vi "niSwitch DMM-array.vi"() -> ()   [LabVIEW 2011]
doc: "I. Description:\n\nThis example demonstrates how to scan a series of channels on a switch module and take measurements with an NI digital multimeter using handshaking. \n\nHANDSHAKING:\nFirst, the DMM is initiated and waits for a digital pulse from the switch before taking any measurements. When the switch scanning task is started, it connects the first channel in its scan list, waits for the channel to settle and generates a digital pulse-Scan Advanced. When the DMM receives this digital pulse, it takes the first measurement and generates a digital pulse-Measurement Complete (MC). When the switch receives this digital pulse, it advances to the next entry in its scan list and this continues.\n\nII. Instructions for Running:\n\nTo make this example work with your switch, complete the following:\nSWITCH SETUP: (refer to the NI Switches Help) \nEnter the DAQmx/traditional DAQ switch resource name.\nSelect the correct topology for your switch module.\nEnter a valid scan list.\nSelect valid values for Trigger Input and Scan Advanced Output. \n\nDMM SETUP: (refer to your NI DMM documentation)\nEnter the DAQmx/traditional DAQ DMM resource name.\nSelect measurement type, range and resolution.\nEnter number of samples.\nSelect a valid Measurement Complete Destination and Trigger Source.\n\nRefer to the NI Switches Help to determine if your switch supports scanning, the scan list syntax, and the valid channel names and valid resource names for your switch module.\n\nIII. Block Diagram Steps:\n\nA) The switch is configured first. Triggers and scan list are set. The scanning configuration is downloaded to the hardware with niSwitch Commit.vi.\nB) The DMM is configured. Functions, range, resolution, triggers and number of points to take are set. When the DMM initiates, it configures its hardware according to the settings and waits for a trigger. \nC) When the switch initiates it connects the first channels in its scan list, waits for the relays to settle and send its Scan Advanced signal to trigger the DMM for its first measurement. Once the DMM has taken a measurement, the DMM sends its MC signal to the switch to advance to the next entry in the scan list. \nD) The DMM returns to the user the number of measurements specified in \"Samples to Fetch at a Time\". When the stop button is pushed the acquisition stops.\nE) Terminates the scanning operation, closes the session to the switch, and displays errors if any.\n\nIV. I/O Connections Overview:\n\nRefer to the NI Switches Getting Started Guide and NI Switches Help for information about connecting signals to your switch module."
uses:
  <instrlib>/niDMM/nidmm.llb/niDMM Function.ctl
  <instrlib>/niSwitch/niSwitch.LLB/niSwitch Topologies.ctl
  <instrlib>/niDMM/nidmm.llb/niDMM Trigger.ctl
  <instrlib>/niDMM/nidmm.llb/niDMM Sample Trigger.ctl
  <vilib>/Utility/NIReport.llb/NI_report.lvclass
  <instrlib>/niDMM/nidmm.llb/niDMM Configure Measurement Absolute.vi
  <vilib>/addons/_office/excel.llb/Excel Easy Table (str).vi
  <vilib>/addons/_office/NI_ReportGenerationToolkit.lvlib
  <vilib>/Utility/NIReport.llb/Excel/NI_Excel.lvclass
panel:
  in  "自低向高色码表":u32[](array[colorbox])=[16860, 5898160, 6745856, 16765184, 16711680]
  out "转置的数组":dbl[][](array[numeric])=[[0.49997470177871867, 0.4999905131670195, 0.4999715395010585, 0.5000284604989416, 0.49999367544467965, 0.5000158113883009, 0.4999873508893593, 0.5, 0.5, 0.499981026334039], [0.5000031622776602, 0.5000126491106407, 0.49997470177871867, 0.4999715395010585, 0.5, 0.5000252982212814, 0.5000031622776602, 0.4999905131670195, 0.49997786405637884, 0.5], [0.5, 0.499981026334039, 0.4999905131670195, 0.5000221359436212, 0.49997470177871867, 0.5000126491106407, 0.49999367544467965, 0.5000221359436212, 0.5000221359436212, 0.499981026334039], [0.5000158113883009, 0.5000252982212814, 0.5000284604989416, 0.4999905131670195, 0.5000284604989416, 0.5000284604989416, 0.5000063245553203, 0.49998418861169913, 0.49998418861169913, 0.5000252982212814], [0.5000221359436212, 0.49997470177871867, 0.49997470177871867, 0.5, 0.5, 0.49997786405637884, 0.5000031622776602, 0.5000063245553203, 0.5000158113883009, 0.500018973665961], [0.4999873508893593, 0.5000063245553203, 0.5000284604989416, 0.49997786405637884, 0.4999715395010585, 0.499981026334039, 0.5000126491106407, 0.49999367544467965, 0.499981026334039, 0.4999968377223398], [0.5000252982212814, 0.5000158113883009, 0.5000158113883009, 0.5000094868329805, 0.4999968377223398, 0.5000221359436212, 0.5000126491106407, 0.5000221359436212, 0.5, 0.4999873508893593], [0.5, 0.500018973665961, 0.49997470177871867, 0.5000094868329805, 0.499981026334039, 0.49998418861169913, 0.49997470177871867, 0.49997470177871867, 0.5000094868329805, 0.5000126491106407], [0.4999873508893593, 0.49998418861169913, 0.5000284604989416, 0.5000126491106407, 0.5000094868329805, 0.5000284604989416, 0.49999367544467965, 0.5, 0.5000221359436212, 0.49999367544467965], [0.500018973665961, 0.4999968377223398, 0.5000221359436212, 0.5000094868329805, 0.5000094868329805, 0.5000031622776602, 0.5000126491106407, 0.49997470177871867, 0.5000158113883009, 0.5000063245553203]]
  in  "选项卡控件":enum32{"强度图", "数据"}(tab)
  in  "Enum":enum16{"最大值", "最小值"}(ring)
  out "强度极限图":dbl[][](graph)=[[0.49997470177871867, 0.4999905131670195, 0.4999715395010585, 0.5000284604989416, 0.49999367544467965, 0.5000158113883009, 0.4999873508893593, 0.5, 0.5, 0.499981026334039], [0.5000031622776602, 0.5000126491106407, 0.49997470177871867, 0.4999715395010585, 0.5, 0.5000252982212814, 0.5000031622776602, 0.4999905131670195, 0.49997786405637884, 0.5], [0.5, 0.499981026334039, 0.4999905131670195, 0.5000221359436212, 0.49997470177871867, 0.5000126491106407, 0.49999367544467965, 0.5000221359436212, 0.5000221359436212, 0.499981026334039], [0.5000158113883009, 0.5000252982212814, 0.5000284604989416, 0.4999905131670195, 0.5000284604989416, 0.5000284604989416, 0.5000063245553203, 0.49998418861169913, 0.49998418861169913, 0.5000252982212814], [0.5000221359436212, 0.49997470177871867, 0.49997470177871867, 0.5, 0.5, 0.49997786405637884, 0.5000031622776602, 0.5000063245553203, 0.5000158113883009, 0.500018973665961], [0.4999873508893593, 0.5000063245553203, 0.5000284604989416, 0.49997786405637884, 0.4999715395010585, 0.499981026334039, 0.5000126491106407, 0.49999367544467965, 0.499981026334039, 0.4999968377223398], [0.5000252982212814, 0.5000158113883009, 0.5000158113883009, 0.5000094868329805, 0.4999968377223398, 0.5000221359436212, 0.5000126491106407, 0.5000221359436212, 0.5, 0.4999873508893593], [0.5, 0.500018973665961, 0.49997470177871867, 0.5000094868329805, 0.499981026334039, 0.49998418861169913, 0.49997470177871867, 0.49997470177871867, 0.5000094868329805, 0.5000126491106407], [0.4999873508893593, 0.49998418861169913, 0.5000284604989416, 0.5000126491106407, 0.5000094868329805, 0.5000284604989416, 0.49999367544467965, 0.5, 0.5000221359436212, 0.49999367544467965], [0.500018973665961, 0.4999968377223398, 0.5000221359436212, 0.5000094868329805, 0.5000094868329805, 0.5000031622776602, 0.5000126491106407, 0.49997470177871867, 0.5000158113883009, 0.5000063245553203]]
  out "强度图":dbl[][](graph)=[[0.49997470177871867, 0.4999905131670195, 0.4999715395010585, 0.5000284604989416, 0.49999367544467965, 0.5000158113883009, 0.4999873508893593, 0.5, 0.5, 0.499981026334039], [0.5000031622776602, 0.5000126491106407, 0.49997470177871867, 0.4999715395010585, 0.5, 0.5000252982212814, 0.5000031622776602, 0.4999905131670195, 0.49997786405637884, 0.5], [0.5, 0.499981026334039, 0.4999905131670195, 0.5000221359436212, 0.49997470177871867, 0.5000126491106407, 0.49999367544467965, 0.5000221359436212, 0.5000221359436212, 0.499981026334039], [0.5000158113883009, 0.5000252982212814, 0.5000284604989416, 0.4999905131670195, 0.5000284604989416, 0.5000284604989416, 0.5000063245553203, 0.49998418861169913, 0.49998418861169913, 0.5000252982212814], [0.5000221359436212, 0.49997470177871867, 0.49997470177871867, 0.5, 0.5, 0.49997786405637884, 0.5000031622776602, 0.5000063245553203, 0.5000158113883009, 0.500018973665961], [0.4999873508893593, 0.5000063245553203, 0.5000284604989416, 0.49997786405637884, 0.4999715395010585, 0.499981026334039, 0.5000126491106407, 0.49999367544467965, 0.499981026334039, 0.4999968377223398], [0.5000252982212814, 0.5000158113883009, 0.5000158113883009, 0.5000094868329805, 0.4999968377223398, 0.5000221359436212, 0.5000126491106407, 0.5000221359436212, 0.5, 0.4999873508893593], [0.5, 0.500018973665961, 0.49997470177871867, 0.5000094868329805, 0.499981026334039, 0.49998418861169913, 0.49997470177871867, 0.49997470177871867, 0.5000094868329805, 0.5000126491106407], [0.4999873508893593, 0.49998418861169913, 0.5000284604989416, 0.5000126491106407, 0.5000094868329805, 0.5000284604989416, 0.49999367544467965, 0.5, 0.5000221359436212, 0.49999367544467965], [0.500018973665961, 0.4999968377223398, 0.5000221359436212, 0.5000094868329805, 0.5000094868329805, 0.5000031622776602, 0.5000126491106407, 0.49997470177871867, 0.5000158113883009, 0.5000063245553203]]
  out "Measurements":dbl[](array[numeric])=[0.499981026334039, 0.5, 0.499981026334039, 0.5000252982212814, 0.500018973665961, 0.4999968377223398, 0.4999873508893593, 0.5000126491106407, 0.49999367544467965, 0.5000063245553203, 0.5, 0.49997786405637884, 0.5000221359436212, 0.49998418861169913, 0.5000158113883009, 0.499981026334039, 0.5, 0.5000094868329805, 0.5000221359436212, 0.5000158113883009, 0.5, 0.4999905131670195, 0.5000221359436212, 0.49998418861169913, 0.5000063245553203, 0.49999367544467965, 0.5000221359436212, 0.49997470177871867, 0.5, 0.49997470177871867, 0.4999873508893593, 0.5000031622776602, 0.49999367544467965, 0.5000063245553203, 0.5000031622776602, 0.5000126491106407, 0.5000126491106407, 0.49997470177871867, 0.49999367544467965, 0.5000126491106407, 0.5000158113883009, 0.5000252982212814, 0.5000126491106407, 0.5000284604989416, 0.49997786405637884, 0.499981026334039, 0.5000221359436212, 0.49998418861169913, 0.5000284604989416, 0.5000031622776602, 0.49999367544467965, 0.5, 0.49997470177871867, 0.5000284604989416, 0.5, 0.4999715395010585, 0.4999968377223398, 0.499981026334039, 0.5000094868329805, 0.5000094868329805, 0.5000284604989416, 0.4999715395010585, 0.5000221359436212, 0.4999905131670195, 0.5, 0.49997786405637884, 0.5000094868329805, 0.5000094868329805, 0.5000126491106407, 0.5000094868329805, 0.4999715395010585, 0.49997470177871867, 0.4999905131670195, 0.5000284604989416, 0.49997470177871867, 0.5000284604989416, 0.5000158113883009, 0.49997470177871867, 0.5000284604989416, 0.5000221359436212, 0.4999905131670195, 0.5000126491106407, 0.499981026334039, 0.5000252982212814, 0.49997470177871867, 0.5000063245553203, 0.5000158113883009, 0.500018973665961, 0.49998418861169913, 0.4999968377223398, 0.49997470177871867, 0.5000031622776602, 0.5, 0.5000158113883009, 0.5000221359436212, 0.4999873508893593, 0.5000252982212814, 0.5, 0.4999873508893593, 0.500018973665961] caption="原始数据" format="%.7f"
  out "输出数组":dbl[][](array[numeric])=[[0.499981026334039, 0.5, 0.499981026334039, 0.5000252982212814, 0.500018973665961, 0.4999968377223398, 0.4999873508893593, 0.5000126491106407, 0.49999367544467965, 0.5000063245553203], [0.5, 0.49997786405637884, 0.5000221359436212, 0.49998418861169913, 0.5000158113883009, 0.499981026334039, 0.5, 0.5000094868329805, 0.5000221359436212, 0.5000158113883009], [0.5, 0.4999905131670195, 0.5000221359436212, 0.49998418861169913, 0.5000063245553203, 0.49999367544467965, 0.5000221359436212, 0.49997470177871867, 0.5, 0.49997470177871867], [0.4999873508893593, 0.5000031622776602, 0.49999367544467965, 0.5000063245553203, 0.5000031622776602, 0.5000126491106407, 0.5000126491106407, 0.49997470177871867, 0.49999367544467965, 0.5000126491106407], [0.5000158113883009, 0.5000252982212814, 0.5000126491106407, 0.5000284604989416, 0.49997786405637884, 0.499981026334039, 0.5000221359436212, 0.49998418861169913, 0.5000284604989416, 0.5000031622776602], [0.49999367544467965, 0.5, 0.49997470177871867, 0.5000284604989416, 0.5, 0.4999715395010585, 0.4999968377223398, 0.499981026334039, 0.5000094868329805, 0.5000094868329805], [0.5000284604989416, 0.4999715395010585, 0.5000221359436212, 0.4999905131670195, 0.5, 0.49997786405637884, 0.5000094868329805, 0.5000094868329805, 0.5000126491106407, 0.5000094868329805], [0.4999715395010585, 0.49997470177871867, 0.4999905131670195, 0.5000284604989416, 0.49997470177871867, 0.5000284604989416, 0.5000158113883009, 0.49997470177871867, 0.5000284604989416, 0.5000221359436212], [0.4999905131670195, 0.5000126491106407, 0.499981026334039, 0.5000252982212814, 0.49997470177871867, 0.5000063245553203, 0.5000158113883009, 0.500018973665961, 0.49998418861169913, 0.4999968377223398], [0.49997470177871867, 0.5000031622776602, 0.5, 0.5000158113883009, 0.5000221359436212, 0.4999873508893593, 0.5000252982212814, 0.5, 0.4999873508893593, 0.500018973665961]]
  in  "error in (no error)":errorcluster caption="错误输入（无错误）"
  in  "Save":bool caption="Stop"
  out "大小":i32=100
  in  "通道个数":i32=100 min=9 max=100
  in  "最大采集时间 (毫秒)":i32=5000
  in  "topology name":T1="2530/1-Wire Dual 64x1 Mux" caption="拓扑名称"
  in  "measurement type":T2=enum."DC Current" caption="测量类型"
  in  "range":dbl=0.5 caption="范围" format="%.2f"
  in  "resolution":dbl=1e-05 caption="分辨率" format="%.0p"
  in  "resource name":refnum<k15>="4071" caption="万用表名称"
  in  "scan list":string="ch0->com0&ch64->com4;ch1->com0&ch64->com4;ch2->com0&ch64->com4;ch3->com0&ch64->com4;ch4->com0&ch64->com4;ch5->com0&ch64->com4;ch6->com0&ch64->com4;ch7->com0&ch64->com4;ch8->com0&ch64->com4;ch9->com0&ch64->com4;ch0->com0&ch65->com4;ch1->com0&ch65->com4;ch2->com0&ch65->com4;ch3->com0&ch65->com4;ch4->com0&ch65->com4;ch5->com0&ch65->com4;ch6->com0&ch65->com4;ch7->com0&ch65->com4;ch8->com0&ch65->com4;ch9->com0&ch65->com4;ch0->com0&ch66->com4;ch1->com0&ch66->com4;ch2->com0&ch66->com4;ch3->com0&ch66->com4;ch4->com0&ch66->com4;ch5->com0&ch66->com4;ch6->com0&ch66->com4;ch7->com0&ch66->com4;ch8->com0&ch66->com4;ch9->com0&ch66->com4;ch0->com0&ch67->com4;ch1->com0&ch67->com4;ch2->com0&ch67->com4;ch3->com0&ch67->com4;ch4->com0&ch67->com4;ch5->com0&ch67->com4;ch6->com0&ch67->com4;ch7->com0&ch67->com4;ch8->com0&ch67->com4;ch9->com0&ch67->com4;ch0->com0&ch68->com4;ch1->com0&ch68->com4;ch2->com0&ch68->com4;ch3->com0&ch68->com4;ch4->com0&ch68->com4;ch5->com0&ch68->com4;ch6->com0&ch68->com4;ch7->com0&ch68->com4;ch8->com0&ch68->com4;ch9->com0&ch68->com4;ch0->com0&ch69->com4;ch1->com0&ch69->com4;ch2->com0&ch69->com4;ch3->com0&ch69->com4;ch4->com0&ch69->com4;ch5->com0&ch69->com4;ch6->com0&ch69->com4;ch7->com0&ch69->com4;ch8->com0&ch69->com4;ch9->com0&ch69->com4;ch0->com0&ch70->com4;ch1->com0&ch70->com4;ch2->com0&ch70->com4;ch3->com0&ch70->com4;ch4->com0&ch70->com4;ch5->com0&ch70->com4;ch6->com0&ch70->com4;ch7->com0&ch70->com4;ch8->com0&ch70->com4;ch9->com0&ch70->com4;\nch0->com0&ch71->com4;ch1->com0&ch71->com4;ch2->com0&ch71->com4;ch3->com0&ch71->com4;ch4->com0&ch71->com4;ch5->com0&ch71->com4;ch6->com0&ch71->com4;ch7->com0&ch71->com4;ch8->com0&ch71->com4;ch9->com0&ch71->com4;ch0->com0&ch72->com4;ch1->com0&ch72->com4;ch2->com0&ch72->com4;ch3->com0&ch72->com4;ch4->com0&ch72->com4;ch5->com0&ch72->com4;ch6->com0&ch72->com4;ch7->com0&ch72->com4;ch8->com0&ch72->com4;ch9->com0&ch72->com4;ch0->com0&ch73->com4;ch1->com0&ch73->com4;ch2->com0&ch73->com4;ch3->com0&ch73->com4;ch4->com0&ch73->com4;ch5->com0&ch73->com4;ch6->com0&ch73->com4;ch7->com0&ch73->com4;ch8->com0&ch73->com4; ch9->com0&ch73->com4;\n" caption="扫描列表"
  in  "resource name":refnum<k15>="Dev2" caption="开关卡名称"
  in  "Stop":bool
  # "开关卡设备"
  # "万用表设备"
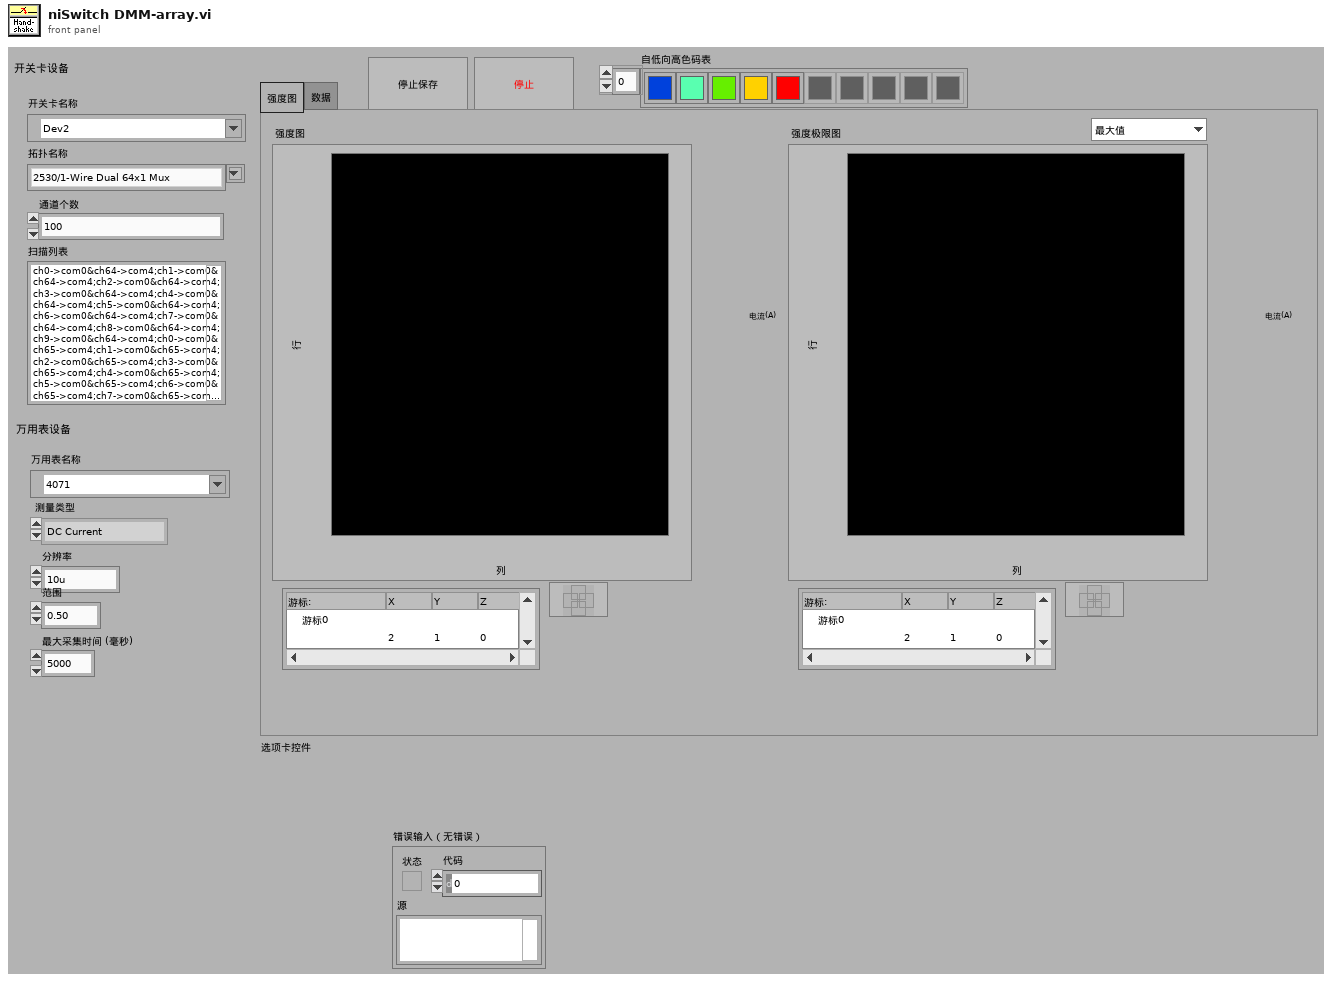
[diagram p1: front panel]
types:
  T1 = typedef "niSwitch Topologies.ctl" = string
  T2 = typedef "niDMM Function.ctl" = enum16{"DC Volts", "AC Volts", "DC Current", "AC Current", "2-wire Resistance", "4-wire Resistance", "Diode", "Frequency", "Period", "AC Volts DC Coupled", "Capacitance", "Inductance", "Temperature"}
  T3 = enum16{"maximized", "minimized", "normal", "no change"}
  T4 = enum16{"Standard Report", "HTML", "Word", "Excel"}
  T5 = typedef "niDMM Trigger.ctl" = enum16{"Immediate", "External", "TTL 0", "TTL 1", "TTL 2", "TTL 3", "TTL 4", "TTL 5", "TTL 6", "Software", "TTL 7", "PXI Star", "LBR Trig 1", "Aux Trig 1"}
  T6 = enum16{"None", "External", "TTL0", "TTL1", "TTL2", "TTL3", "TTL4", "TTL5", "TTL6", "TTL7", "ECL0", "ECL1", "PXI Star", "Rear Connector", "Front Connector", "Rear Connector Module 1", "Rear Connector Module 2", "Rear Connector Module 3", "Rear Connector Module 4", "Rear Connector Module 5", "Rear Connector Module 6", "Rear Connector Module 7", "Rear Connector Module 8", "Rear Connector Module 9", "Rear Connector Module 10", "Rear Connector Module 11", "Rear Connector Module 12", "Front Connector Module 1", "Front Connector Module 2", "Front Connector Module 3", "Front Connector Module 4", "Front Connector Module 5", "Front Connector Module 6", "Front Connector Module 7", "Front Connector Module 8", "Front Connector Module 9", "Front Connector Module 10", "Front Connector Module 11", "Front Connector Module 12"}
  T7 = enum16{"Immediate", "External", "TTL0", "TTL1", "TTL2", "TTL3", "TTL4", "TTL5", "TTL6", "TTL7", "ECL0", "ECL1", "PXI Star", "Software Trigger Function", "Rear Connector", "Front Connector", "Rear Connector of Module 1", "Rear Connector of Module 2", "Rear Connector of Module 3", "Rear Connector of Module 4", "Rear Connector of Module 5", "Rear Connector of Module 6", "Rear Connector of Module 7", "Rear Connector of Module 8", "Rear Connector of Module 9", "Rear Connector of Module 10", "Rear Connector of Module 11", "Rear Connector of Module 12", "Front Connector of Module 1", "Front Connector of Module 2", "Front Connector of Module 3", "Front Connector of Module 4", "Front Connector of Module 5", "Front Connector of Module 6", "Front Connector of Module 7", "Front Connector of Module 8", "Front Connector of Module 9", "Front Connector of Module 10", "Front Connector of Module 11", "Front Connector of Module 12"}
  T8 = typedef "niDMM Sample Trigger.ctl" = enum16{"Immediate", "External", "TTL 0", "TTL 1", "TTL 2", "TTL 3", "TTL 4", "TTL 5", "TTL 6", "Interval", "Software", "TTL 7", "PXI Star", "LBR Trig 1", "Aux Trig 1"}
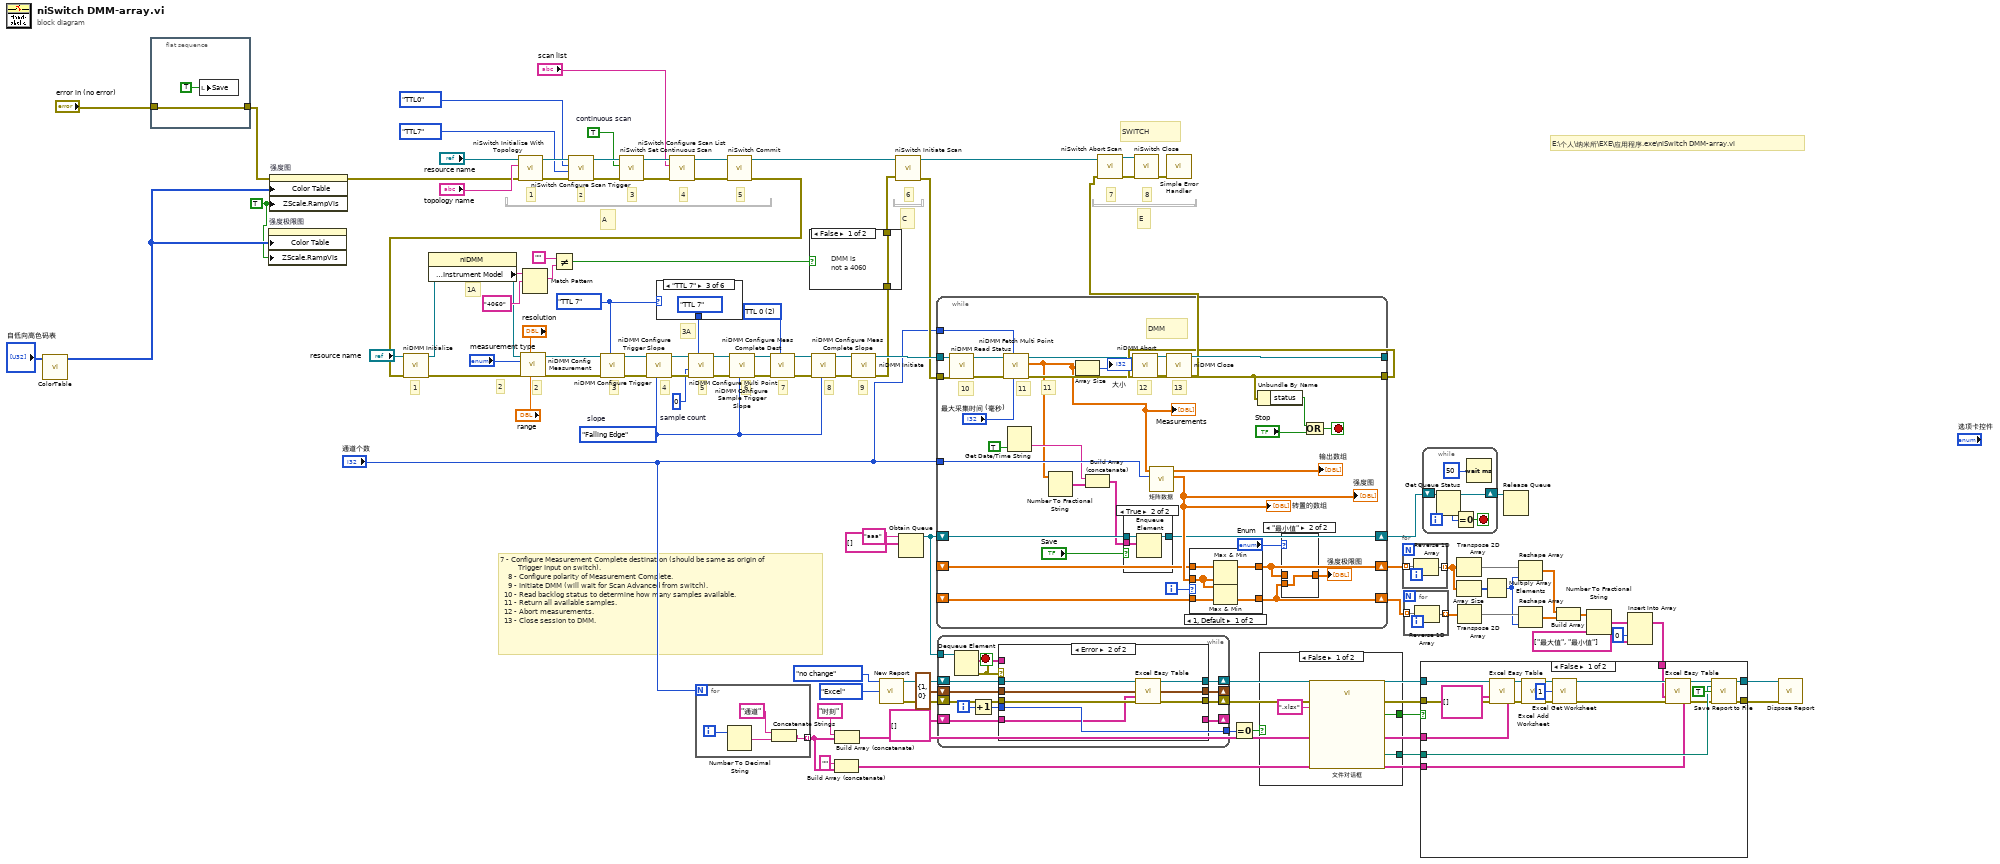
[diagram p0: block diagram]
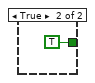
[diagram p2: hidden frame]
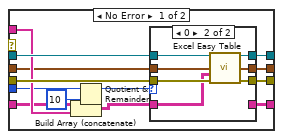
[diagram p4: hidden frame]
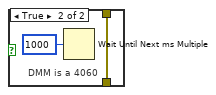
[diagram p9: hidden frame]
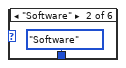
[diagram p11: hidden frame]
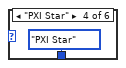
[diagram p12: hidden frame]
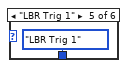
[diagram p13: hidden frame]
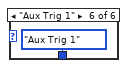
[diagram p14: hidden frame]
diagram:
  w58 = niDMM_Trigger."TTL 7" ("trigger source")
  w73 = u16 2 items=["None", "External", "TTL 0", "TTL 1", "TTL 2", "TTL 3", "TTL 4", "TTL 5", "TTL 6", "TTL 7", "LBR Trig 0"] ("measurement complete destination")
  w2 = TRUE ("Z标尺.颜色梯度可见")
  w68 = enum16{"Rising Edge", "Falling Edge"}."Falling Edge"  # slope
  w84 = 0  # sample count
  w102 = TRUE  # continuous scan
  # "E:\\个人\\纳米所\\EXE\\应用程序.exe\\niSwitch DMM-array.vi"
  # "2"
  # "5"
  # "7 - Configure Measurement Complete destination (should be same as origin of\n         Trigger Input on switch).\n    8 - Configure polarity of Measurement Complete.\n    9 - Initiate DMM (will wait for Scan Advanced from switch).\n  10 - Read backlog status to determine how many samples available.  \n  11 - Return all available samples.\n  12 - Abort measurements.\n  13 - Close session to DMM."
  # "9"
  # "13"
  # "12"
  # "8"
  # "3A"
  # "1A"
  # "4"
  # "6"
  # "11"
  # "5"
  # "7"
  # "3"
  # "2"
  # "1"
  # "E"
  # "C"
  # "A"
  # "DMM"
  # "SWITCH"
  # "6"
  # "8"
  # "7"
  # "4"
  # "3"
  # "2"
  # "1"
  n1 = call "ColorTable.vi"("色码表"="自低向高色码表") -> ("数组"=w3:u32[])  [unwired: 10 in]
  n2 = flat-sequence {
    tunnel: "error in (no error)" -> [w107]
    tunnel: [w107] -> w44
    frame #0 {
      n3 = local write "Save"(TRUE ("Save")) -> ()
    }
  }
  n4 = property on="强度极限图" class="IntGraph (strict)"("Color Table"=w3, "ZScale.RampVis"=w2) -> ()  [unwired: 2 in, 2 out]
  n5 = property on="强度图" class="IntGraph (strict)"(error in=w44, "Color Table"=w3, "ZScale.RampVis"=w2) -> (error out=w49:errorcluster)  [unwired: 1 in, 1 out]
  n6 = call <instrlib>:"niSwitch Initialize With Topology.vi"("error in (no error)"=w49, "topology name"="topology name", "resource name"="resource name") -> ("error out"=w98:errorcluster, "instrument handle out"=w99:refnum<k15>)  [unwired: 7 in]
  n7 = call <instrlib>:"niSwitch Configure Scan Trigger.vi"("error in (no error)"=w98, "scan advanced output (External)"=T6."TTL7" ("scan advanced output"), "trigger input (External)"=T7."TTL0" ("trigger input"), "instrument handle"=w99) -> ("error out"=w103:errorcluster, "instrument handle out"=w105:refnum<k15>)  [unwired: 6 in]
  n8 = call <instrlib>:"niSwitch Set Continuous Scan.vi"("error in (no error)"=w103, "continuous scan (False)"=w102, "instrument handle"=w105) -> ("error out"=w96:errorcluster, "instrument handle out"=w97:refnum<k15>)  [unwired: 7 in]
  n9 = case shown="\"TTL 7\"" w58 {
    selector: w58 -> [w109 _ _ _ _ _]
    tunnel: [w109 niDMM_Sample_Trigger."Software" ("Sample Trigger") niDMM_Sample_Trigger."TTL 7" ("Sample Trigger") niDMM_Sample_Trigger."PXI Star" ("Sample Trigger") niDMM_Sample_Trigger."LBR Trig 1" ("Sample Trigger") niDMM_Sample_Trigger."Aux Trig 1" ("Sample Trigger")] -> w82
    frame "Immediate", Default {
    }
    frame "Software" {
    }
    frame "TTL 7" {
    }
    frame "PXI Star" {
    }
    frame "LBR Trig 1" {
    }
    frame "Aux Trig 1" {
    }
  }
  n10 = call <instrlib>:"niSwitch Configure Scan List.vi"("error in (no error)"=w96, "scan list"="scan list", "instrument handle"=w97) -> ("error out"=w62:errorcluster, "instrument handle out"=w61:refnum<k15>)  [unwired: 7 in]
  n11 = for {
    N: "通道个数" -> [_]
    tunnel: [w115] -> w16 mode=indexing
    i -> [w118]
    n12 = Number To Decimal String(number=w118) -> (decimal integer string=w117:string)  [unwired: 1 in]
    n13 = Concatenate Strings("通道" ("字符串"), w117) -> (w115:string)
  }
  n14 = call <instrlib>:"niSwitch Commit.vi"("error in (no error)"=w62, "instrument handle"=w61) -> ("error out"=w60:errorcluster, "instrument handle out"=w59:refnum<k15>)  [unwired: 8 in]
  n15 = call <instrlib>:"niDMM Initialize.vi"("error in (no error)"=w60, "Instrument Descriptor"="resource name") -> ("error out"=w54:errorcluster, "instrument handle out"=w64:refnum<k15>)  [unwired: 8 in]
  n16 = property class="niDMM"(reference=w64) -> (reference out=w57:refnum<k15>, "Inherent IVI Attributes:Instrument Identification:Instrument Model"=w65:string)  [unwired: 1 in, 1 out]
  n17 = call-poly <instrlib>:"niDMM Config Measurement.vi"("Range"="range", "Resolution"="resolution", "error in (no error)"=w54, "Function"="measurement type", "instrument handle"=w57) -> ("error out"=w51:errorcluster, "instrument handle out"=w52:refnum<k15>)  [unwired: 5 in]
  n18 = Match Pattern(string=w65, regular expression="4060") -> (match substring=w79:string)  [unwired: 1 in, 3 out]
  n19 = Not Equal?(x="", y=w79) -> (x != y?=w77:bool)
  n20 = call <instrlib>:"niDMM Configure Trigger.vi"("Trigger Source"=w58, "error in (no error)"=w51, "instrument handle"=w52) -> ("error out"=w89:errorcluster, "instrument handle out"=w90:refnum<k15>)  [unwired: 7 in]
  n21 = call <instrlib>:"niDMM Configure Trigger Slope.vi"("Slope"=w68, "error in (no error)"=w89, "instrument handle"=w90) -> ("error out"=w87:errorcluster, "instrument handle out"=w88:refnum<k15>)  [unwired: 7 in]
  n22 = call <instrlib>:"niDMM Configure Multi Point.vi"("Sample Trigger"=w82, "error in (no error)"=w87, "Sample Count"=w84, "instrument handle"=w88) -> ("error out"=w85:errorcluster, "instrument handle out"=w86:refnum<k15>)  [unwired: 6 in]
  n23 = call <instrlib>:"niDMM Configure Sample Trigger Slope.vi"("Slope"=w68, "error in (no error)"=w85, "instrument handle"=w86) -> ("error out"=w75:errorcluster, "instrument handle out"=w74:refnum<k15>)  [unwired: 7 in]
  n24 = call <instrlib>:"niDMM Configure Meas Complete Dest.vi"("Measurement Complete Destination"=w73, "error in (no error)"=w75, "instrument handle"=w74) -> ("error out"=w69:errorcluster, "instrument handle out"=w72:refnum<k15>)  [unwired: 7 in]
  n25 = call <instrlib>:"niDMM Configure Meas Complete Slope.vi"("Slope"=w68, "error in (no error)"=w69, "instrument handle"=w72) -> ("error out"=w70:errorcluster, "instrument handle out"=w71:refnum<k15>)  [unwired: 7 in]
  n26 = Build Array (concatenate)("", w16) -> (w14:string[])
  n27 = Build Array (concatenate)("时刻", w16) -> (w8:string[])
  n28 = call <instrlib>:"niDMM Initiate.vi"("error in (no error)"=w70, "instrument handle"=w71) -> ("error out"=w81:errorcluster, "instrument handle out"=w94:refnum<k15>)  [unwired: 8 in]
  n29 = case shown="False" w77 {
    tunnel: w81 -> [w119 w120]
    tunnel: [w119 w120] -> w76
    frame False {
      # "DMM is \nnot a 4060"
    }
    frame True {
      # "DMM is a 4060"
      n30 = Wait Until Next ms Multiple(millisecond multiple=u32 1000) -> ()  [unwired: 1 out]
    }
  }
  n31 = call <vilib>:"New Report.vi"("window state (normal)"=T3."no change", "report type"=T4."Excel") -> ("report out"=w39:refnum<class "NI_report.lvclass">, "error out"=w38:errorcluster)  [unwired: 12 in]
  n32 = call <instrlib>:"niSwitch Initiate Scan.vi"("error in (no error)"=w76, "instrument handle"=w59) -> ("error out"=w47:errorcluster, "instrument handle out"=w95:refnum<k15>)  [unwired: 8 in]
  n33 = Obtain Queue(name (unnamed)="aaa", element data type=string[] []) -> (queue out=w37:refnum<queue>)  [unwired: 3 in, 2 out]
  n34 = while {
    tunnel: [w151] -> w83
    tunnel: w94 -> [w147]
    tunnel: [w150] -> w46
    tunnel: w47 -> [w144]
    tunnel: "通道个数" -> [w141]
    tunnel: "通道个数" -> [w139]
    shift-right: [w129] -> w27
    shift-left: _ -> [w132]
    shift-right: [w128] -> w25
    shift-left: _ -> [w131]
    shift-right: [w124] -> w7
    shift-left: w37 -> [w126]
    i -> [w134]
    stop <- w142 stop-if-true
    # "11"
    # "10"
    # "9"
    n35 = call <instrlib>:"niDMM Read Status.vi"("error in (no error)"=w144, "instrument handle"=w147) -> ("error out"=w146:errorcluster, "instrument handle out"=w145:refnum<k15>)  [unwired: 6 in, 2 out]
    n36 = call <instrlib>:"niDMM Fetch Multi Point.vi"("Maximum Time (msec)"="最大采集时间 (毫秒)", "Number to Fetch"=w139, "error in (no error)"=w146, "instrument handle"=w145) -> ("error out"=w150:errorcluster, "Measurements"=w122:dbl[], "instrument handle out"=w151:refnum<k15>)  [unwired: 4 in, 1 out]
    "Measurements" <- w122
    n37 = Get Date/Time String(want seconds? (F)=TRUE ("需要秒？(F)")) -> (time string=w138:string)  [unwired: 2 in, 1 out]
    n38 = Number To Fractional String(number=w122) -> (F-format string=w137:string[])  [unwired: 3 in]
    n39 = Array Size(array=w122) -> (size(s)=→"大小":i32)
    n40 = Build Array (concatenate)(w138, w137) -> (w125:string[])
    n41 = case shown="True" "Save" {
      tunnel: w126 -> [w152 w155]
      tunnel: w125 -> [_ w154]
      tunnel: [w152 w153] -> w124
      frame False {
      }
      frame True {
        n42 = Enqueue Element(queue=w155, element=w154) -> (queue out=w153:refnum<queue>)  [unwired: 2 in, 2 out]
      }
    }
    n43 = call "矩阵数据.vi"("数值"=w141, "数据"=w122) -> ("强度矩阵"=w133:dbl[][], "原始矩阵"=→"输出数组":dbl[][])  [unwired: 8 in]
    "强度图" <- w133
    "转置的数组" <- w133
    n44 = case shown="1, Default" w134 {
      tunnel: w133 -> [w160 w163]
      tunnel: [w161 w163] -> w129
      tunnel: [w158 w163] -> w128
      tunnel: w132 -> [w162 _]
      tunnel: w131 -> [w159 _]
      frame 1, Default {
        n45 = Max & Min(x=w162, y=w160) -> (max(x,y)=w161:dbl[][])  [unwired: 1 out]
        n46 = Max & Min(x=w160, y=w159) -> (min(x,y)=w158:dbl[][])  [unwired: 1 out]
      }
      frame 0 {
      }
    }
    n47 = Unbundle By Name(w150) -> ("status"=w149:bool)
    n48 = case shown="\"最小值\"" "Enum" {
      tunnel: w129 -> [w156 _]
      tunnel: w128 -> [_ w157]
      tunnel: [w156 w157] -> w127
      frame "最大值", Default {
      }
      frame "最小值" {
      }
    }
    "强度极限图" <- w127
    n49 = Or(x=w149, y="Stop") -> (x .or. y?=w142:bool)
  }
  n50 = while {
    tunnel: w37 -> [w174]
    tunnel: [w166] -> w34
    shift-right: [w170] -> w28
    shift-left: w38 -> [w175]
    shift-right: [w171] -> w29
    shift-left: w39 -> [w176]
    shift-right: [w168] -> _
    shift-left: string[][] [] -> [w167]
    shift-right: [w165] -> _
    shift-left: cluster{"row":i32, "column":i32} {"row"=1, "column"=0} ("next cell bottom-left") -> [w164]
    i -> [w169]
    stop <- w172 stop-if-true
    n51 = Dequeue Element(queue=w174) -> (element=w173:string[], error out=w172:errorcluster)  [unwired: 2 in, 2 out]
    n52 = Increment(x=w169) -> (x+1=w166:i32)
    n53 = case shown="Error" w172 {
      tunnel: w176 -> [w189 w207]
      tunnel: w175 -> [w188 w205]
      tunnel: w173 -> [w187 _]
      tunnel: [w186 w206] -> w171
      tunnel: [w185 w204] -> w170
      tunnel: w166 -> [w180 _]
      tunnel: [w182 _] -> w168
      tunnel: w167 -> [w181 w203]
      tunnel: [w178 w202] -> w165
      tunnel: w164 -> [w177 w201]
      frame No Error {
        n54 = Build Array (concatenate)(w181, w187) -> (w183:string[][])
        n55 = Quotient & Remainder(x=w180, y=10) -> (x-y*floor(x/y)=w184:i32)  [unwired: 1 out]
        n56 = case shown="0" w184 {
          tunnel: w189 -> [w193 w200]
          tunnel: w188 -> [w192 w199]
          tunnel: [w193 w198] -> w186
          tunnel: [w192 w197] -> w185
          tunnel: w183 -> [w191 w196]
          tunnel: [w191 _] -> w182
          tunnel: [w190 w195] -> w178
          tunnel: w177 -> [w190 w194]
          frame 1, Default {
          }
          frame 0 {
            n57 = call-poly <vilib>:"Excel Easy Table.vi"("report in"=w200, "start (0, 0)"=w194, "text data"=w196, "error in (no error)"=w199) -> ("report out"=w198:refnum<class "NI_report.lvclass">, "next cell bottom-left"=w195:cluster{"row":i32, "column":i32}, "error out"=w197:errorcluster)  [unwired: 7 in, 2 out]
          }
        }
      }
      frame Error {
        n58 = call-poly <vilib>:"Excel Easy Table.vi"("report in"=w207, "start (0, 0)"=w201, "text data"=w203, "error in (no error)"=w205) -> ("report out"=w206:refnum<class "NI_report.lvclass">, "next cell bottom-left"=w202:cluster{"row":i32, "column":i32}, "error out"=w204:errorcluster)  [unwired: 7 in, 2 out]
      }
    }
  }
  n59 = call <instrlib>:"niDMM Abort.vi"("error in (no error)"=w46, "instrument handle"=w83) -> ("error out"=w92:errorcluster, "instrument handle out"=w93:refnum<k15>)  [unwired: 8 in]
  n60 = call <instrlib>:"niDMM Close.vi"("error in (no error)"=w92, "instrument handle"=w93) -> ("error out"=w63:errorcluster)  [unwired: 9 in]
  n61 = call <instrlib>:"niSwitch Abort Scan.vi"("error in (no error)"=w63, "instrument handle"=w95) -> ("error out"=w101:errorcluster, "instrument handle out"=w104:refnum<k15>)  [unwired: 8 in]
  n62 = call <instrlib>:"niSwitch Close.vi"("error in (no error)"=w101, "instrument handle"=w104) -> ("error out"=w106:errorcluster)  [unwired: 9 in]
  n63 = call <vilib>:"Simple Error Handler.vi"("error in (no error)"=w106) -> ()  [unwired: 4 in, 5 out]
  n64 = Equal To 0?(x=w34) -> (x = 0?=w9:bool)
  n65 = case shown="False" w9 {
    tunnel: [w209 TRUE ("cancelled")] -> w32
    tunnel: [w208 _] -> w30
    frame False {
      n66 = call "文件对话框"("pattern (all files)"=".xlsx") -> ("selected path"=w208:path, "cancelled"=w209:bool)  [unwired: 11 in, 2 out]
    }
    frame True {
    }
  }
  n67 = for {
    tunnel: w27 -> [w213] mode=indexing
    tunnel: [w212] -> w23 mode=indexing
    n68 = Reverse 1D Array(array=w213) -> (reversed array=w212:dbl[])
  }
  n69 = for {
    tunnel: w25 -> [w215] mode=indexing
    tunnel: [w214] -> w26 mode=indexing
    n70 = Reverse 1D Array(array=w215) -> (reversed array=w214:dbl[])
  }
  n71 = while {
    shift-right: [w219] -> w6
    shift-left: w7 -> [w220]
    stop <- w218 stop-if-true
    n72 = Get Queue Status(queue=w220) -> (queue out=w219:refnum<queue>, # elements in queue=w217:i32)  [unwired: 2 in, 6 out]
    n73 = Equal To 0?(x=w217) -> (x = 0?=w218:bool)
    n74 = Wait (ms)(milliseconds to wait=u32 50) -> ()  [unwired: 1 out]
  }
  n75 = Transpose 2D Array(2D array=w23) -> (transposed array=w24:dbl[][])
  n76 = Array Size(array=w23) -> (size(s)=w22:i32[])
  n77 = Transpose 2D Array(2D array=w26) -> (transposed array=w21:dbl[][])
  n78 = Multiply Array Elements(1:w22) -> (0:w20:i32)
  n79 = Release Queue(queue=w6) -> ()  [unwired: 2 in, 3 out]
  n80 = Reshape Array(w24, w20) -> (w19:dbl[])
  n81 = Reshape Array(w21, w20) -> (w18:dbl[])
  n82 = Build Array(w19, w18) -> (w17:dbl[][])
  n83 = Number To Fractional String(number=w17) -> (F-format string=w12:string[][])  [unwired: 3 in]
  n84 = Insert Into Array(array=w12, index (col)=0 ("disabled index (col)"), new element=string[] ["最大值", "最小值"] ("new element/subarray")) -> (w13:string[][])  [unwired: 1 in]
  n85 = case shown="False" w32 {
    tunnel: [w239 w240] -> w31
    tunnel: [w238 w241] -> w33
    tunnel: w29 -> [w226 w241]
    tunnel: w28 -> [w224 w240]
    tunnel: w30 -> [w236 _]
    tunnel: w13 -> [w228 _]
    tunnel: w14 -> [w227 _]
    tunnel: w8 -> [w222 _]
    frame False {
      n86 = call-poly <vilib>:"Excel Easy Table.vi"("report in"=w226, "text data"=string[][] [], "error in (no error)"=w224, "column headers"=w222) -> ("report out"=w225:refnum<class "NI_report.lvclass">, "error out"=w223:errorcluster)  [unwired: 7 in, 3 out]
      n87 = call <vilib>:"Excel Add Worksheet.vi"("report in"=w225, "error in (no error)"=w223) -> ("report out"=w232:refnum<class "NI_report.lvclass">, "error out"=w231:errorcluster)  [unwired: 12 in]
      n88 = call <vilib>:"Excel Get Worksheet.vi"("report in"=w232, "worksheet index (0)"=1, "error in (no error)"=w231) -> ("report out"=w233:refnum<class "NI_report.lvclass">, "error out"=w229:errorcluster)  [unwired: 11 in]
      n89 = call-poly <vilib>:"Excel Easy Table.vi"("report in"=w233, "text data"=w228, "error in (no error)"=w229, "column headers"=w227) -> ("report out"=w235:refnum<class "NI_report.lvclass">, "error out"=w234:errorcluster)  [unwired: 7 in, 3 out]
      n90 = call-dynamic "Save Report to File.vi"("report in"=w235, "report file path"=w236, "prompt to replace? (F)"=TRUE, "error in (no error)"=w234) -> ("report out"=w238:refnum<class "NI_report.lvclass">, "error out"=w239:errorcluster)  [unwired: 10 in]
    }
    frame True {
    }
  }
  n91 = call-dynamic "Dispose Report.vi"("report in"=w33, "error in (no error)"=w31) -> ()  [unwired: 13 in, 1 out]
